vi "mqttCmdAcknowledge.vi"(0 "_mqtt in":refnum<class "BaseMqttMsg.lvclass">, 11 "error in (no error)":errorcluster) -> (4 "_mqtt out":refnum<class "BaseMqttMsg.lvclass">, 8 "notification":T1, 15 "error out":errorcluster)   [LabVIEW 2020, in "BaseMqttMsg.lvclass"]
uses:
  BaseMqttMsg.lvclass
  mqttTypedef/mqttRXdataCluster.ctl
  mqttTypedef/mqttFixedHeaderResponse.ctl
  mqttTypedef/mqttQOSlevel.ctl
  mqttTypedef/mqttMessageType.ctl
  MQTT Client.lvclass
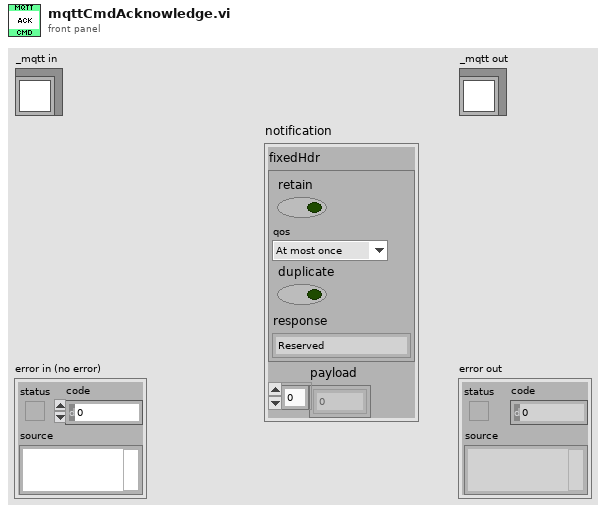
[diagram p1: front panel]
types:
  T1 = typedef "MQTT Client.lvclass/mqttRXdataCluster.ctl" = cluster{"fixedHdr":T2, "payload":u8[]}
  T2 = typedef "MQTT Client.lvclass/mqttFixedHeaderResponse.ctl" = cluster{"retain":bool, "qos":T3, "duplicate":bool, "response":T4}
  T3 = typedef "MQTT Client.lvclass/mqttQOSlevel.ctl" = enum8{"At most once", "At least once", "Exactly once", "Reserved"}
  T4 = typedef "MQTT Client.lvclass/mqttMessageType.ctl" = enum32{"Reserved", "CONNECT", "CONNACK", "PUBLISH", "PUBACK", "PUBREC", "PUBREL", "PUBCOMP", "SUBSCRIBE", "SUBACK", "UNSUBSCRIBE", "UNSUBACK", "PINGREQ", "PINGRESP", "DISCONNECT", "Reserved2"}
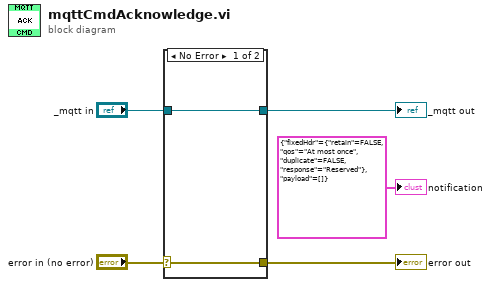
[diagram p0: block diagram]
diagram:
  n1 = case shown="No Error" "error in (no error)" {
    selector: "error in (no error)" -> [w6 w9]
    tunnel: [w6 w9] -> w4
    tunnel: [w7 w8] -> w2
    tunnel: "_mqtt in" -> [w7 w8]
    frame No Error {
    }
    frame Error {
    }
  }
  "error out" <- w4
  "_mqtt out" <- w2
  "notification" <- T1 {"fixedHdr"={"retain"=FALSE, "qos"=enum."At most once", "duplicate"=FALSE, "response"=enum."Reserved"}, "payload"=[]} ("notification")
